vi "Raise Injection Event.vi"(0 "Raiser Name":string, 5 "Raiser Id":string, 7 "Send Injection":bool=TRUE, 9 "Injected Command Directors":refnum<class "CommandDirector.lvclass">[](array[class]), 11 "error in (no error)":errorcluster) -> (15 "error out":errorcluster)   [LabVIEW 2023, in "HAF.lvlib"]
doc: "Helper member to raise an Injection Event if the passed boolean is True. It is always sent as normal priority."
uses:
  HAF.lvlib
  Event Data.ctl
  <vilib>/event_ctls.llb/usereventprio.ctl
  Global Resources.vi
  CommandDirector/CommandDirector.lvclass
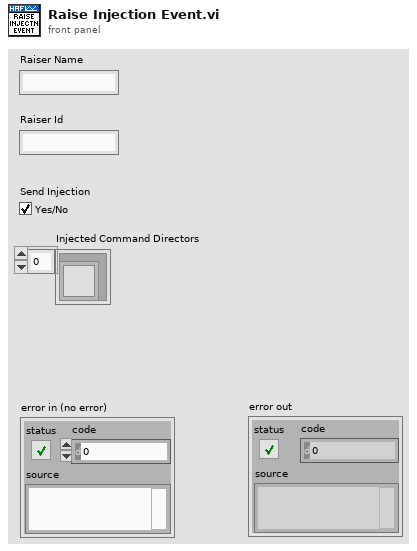
[diagram p1: front panel]
types:
  T1 = typedef "usereventprio.ctl" = enum32{"high priority", "normal priority"}
  T2 = typedef "HAF.lvlib/Event Data.ctl" = cluster{"Raiser Name":string, "Raiser Id":string, "Event Data":variant}
  T3 = typedef "HAF.lvlib/All Events.ctl" = cluster{"Stop":T4, "Pause":T5, "Resume":T6, "Done":T7, "Injection":T8}
  T4 = typedef "HAF.lvlib/Stop Event.ctl" = refnum<user-event>
  T5 = typedef "HAF.lvlib/Pause Event.ctl" = refnum<user-event>
  T6 = typedef "HAF.lvlib/Resume Event.ctl" = refnum<user-event>
  T7 = typedef "HAF.lvlib/Done Event.ctl" = refnum<user-event>
  T8 = typedef "HAF.lvlib/Injection Event.ctl" = refnum<user-event>
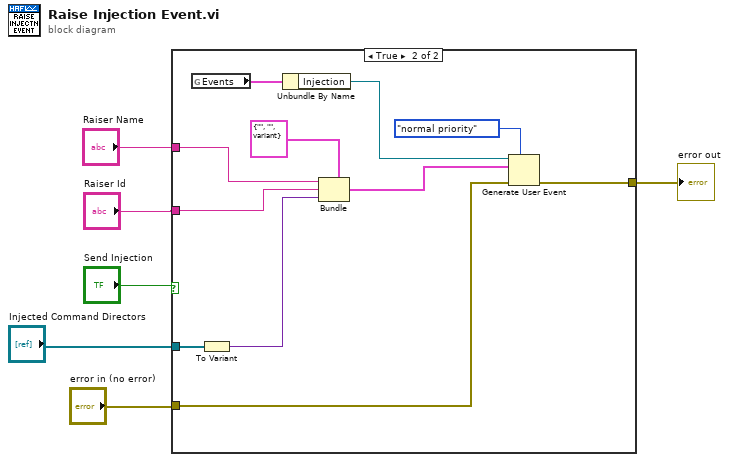
[diagram p0: block diagram]
diagram:
  n1 = case shown="True" "Send Injection" {
    tunnel: "error in (no error)" -> [w7 w14]
    tunnel: "Raiser Name" -> [_ w17]
    tunnel: "Raiser Id" -> [_ w16]
    tunnel: [w7 w13] -> w2
    tunnel: "Injected Command Directors" -> [_ w9]
    frame False {
    }
    frame True {
      n2 = global read "Global Resources.vi" "Events"() -> (w11:T3)
      n3 = To Variant(anything=w9) -> (Variant=w8:variant)
      n4 = Unbundle By Name(w11) -> ("Injection"=w10:T8)
      n5 = Bundle(cluster=T2 {"Raiser Name"="", "Raiser Id"="", "Event Data"=variant} ("Event Data Structure"), "Raiser Name"=w17, "Raiser Id"=w16, "Event Data"=w8) -> (w15:T2)
      n6 = Generate User Event(priority (normal)=usereventprio."normal priority", user event=w10, event data cluster=w15, error in=w14) -> (error out=w13:errorcluster)  [unwired: 1 out]
    }
  }
  "error out" <- w2
